vi "draw a complex line.vi"(6 "number of  grid points":i32=20, 9 "to":cdb=-1.0+1.0i, 11 "from":cdb) -> (3 "array out":cluster{dbl[], dbl[]}[](array[cluster]))   [LabVIEW 2020]
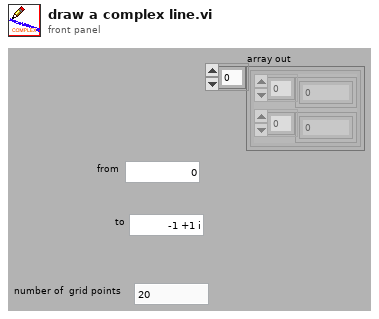
[diagram p1: front panel]
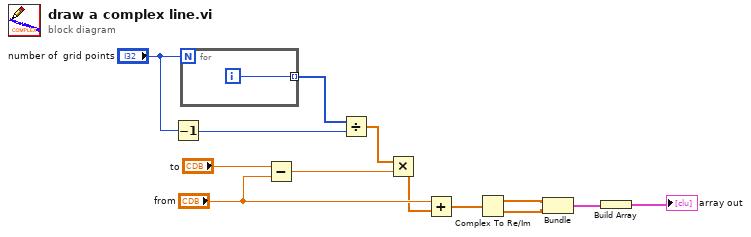
[diagram p0: block diagram]
diagram:
  n1 = Decrement(x="number of  grid points") -> (x-1=w4:i32)
  n2 = for {
    N: "number of  grid points" -> [_]
    tunnel: [w14] -> w5 mode=indexing
    i -> [w14]
  }
  n3 = Subtract(x="to", y="from") -> (x-y=w11:cdb)
  n4 = Divide(x=w5, y=w4) -> (x/y=w3:dbl[])
  n5 = Multiply(x=w3, y=w11) -> (x*y=w10:cdb[])
  n6 = Add(x="from", y=w10) -> (x+y=w9:cdb[])
  n7 = Complex To Re/Im(x + iy=w9) -> (x=w8:dbl[], y=w7:dbl[])
  n8 = Bundle(w8, w7) -> (w2:cluster{dbl[], dbl[]})  [unwired: 1 in]
  n9 = Build Array(w2) -> (→"array out":cluster{dbl[], dbl[]}[])
